vi "SRRead.vi"(8 "error in (no error)":errorcluster, 11 "Data In":T1) -> (0 "error out":errorcluster, 1 "BarCodeRead":string="TH-55ES630W,%71234567,4717523005417\r", 3 "Data Out":T1)   [LabVIEW 2014]
uses:
  controls/Data.ctl
panel:
  out "Boolean":bool
  # "日期"
  # "機種名稱"
  # "機種代號"
  # "商品條碼"
  # "台"
  # "OK"
  # "NG"
  # "台"
  # "總計"
  # "台"
  # "日期"
  # "機種名稱"
  # "機種代號"
  # "商品條碼"
  # "台"
  # "OK"
  # "NG"
  # "台"
  # "總計"
  # "台"
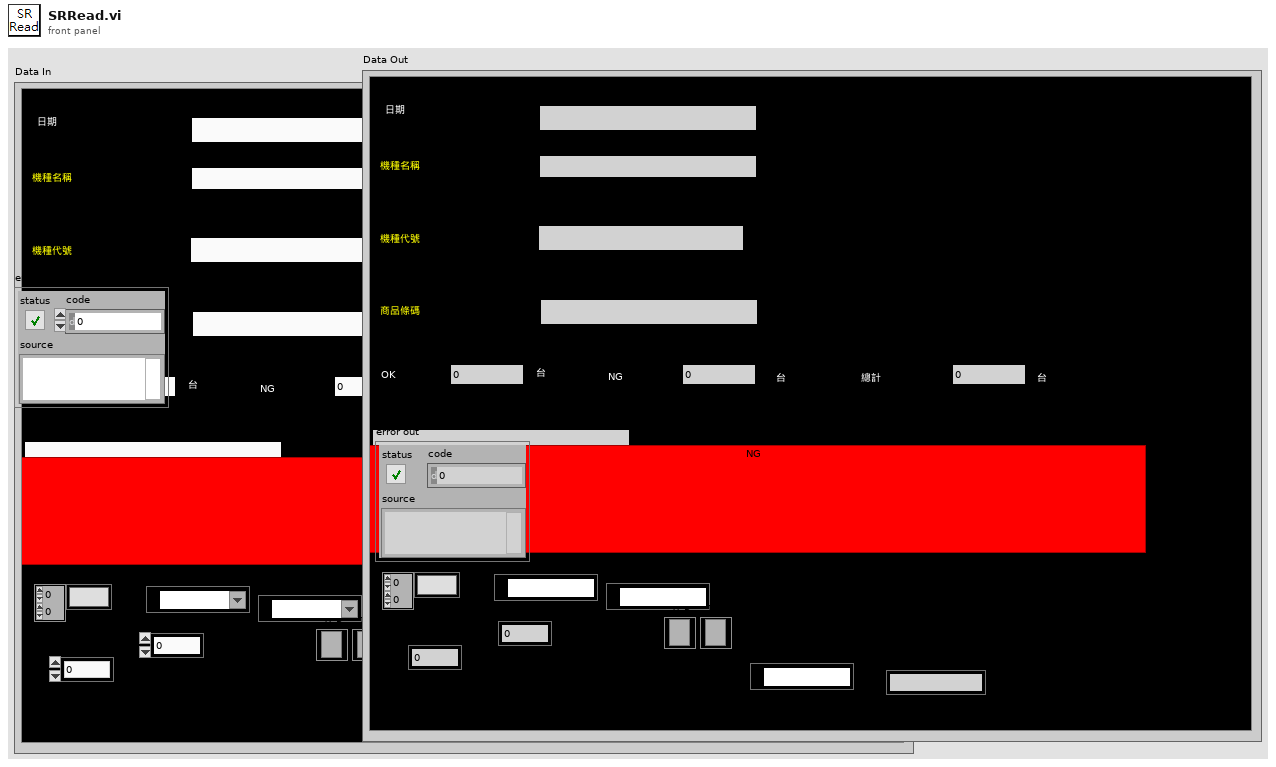
[diagram p1: front panel]
types:
  T1 = typedef "Data.ctl" = cluster{"Date":string, "BarCode1":string, "BarCode2":string, "BarCode3":string, "Message":string, "OK Count":u16, "NG Count":u16, "Total Count":u16, "ModelData":string[][], "OK&NG":bool, "COM1":refnum<visa-resource-name>, "COM2":refnum<visa-resource-name>, "IO":i32, "Time":u32, "TCP":refnum<k5>, "TCP 2":refnum<k5>, "COM3":refnum<visa-resource-name>, "CheckPars":string}
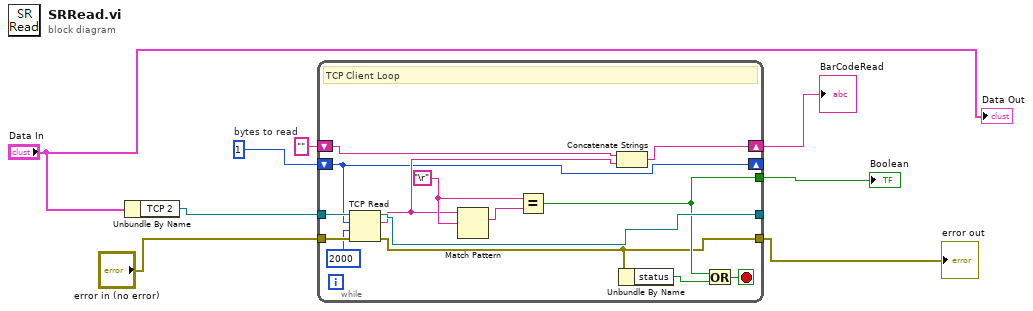
[diagram p0: block diagram]
diagram:
  w8 = 1  # bytes to read
  n1 = Unbundle By Name("Data In") -> ("TCP 2"=w4:refnum<k5>)
  n2 = while {
    tunnel: "error in (no error)" -> [w21]
    tunnel: w4 -> [w22]
    tunnel: [w16] -> _
    tunnel: [w10] -> w2
    shift-right: [w11] -> _
    shift-left: w8 -> [w11]
    tunnel: [w15] -> w7
    shift-right: [w13] -> w5
    shift-left: "" -> [w12]
    stop <- w20 stop-if-true
    w17 = "\r"
    # "TCP Client Loop"
    n3 = TCP Read(connection ID=w22, bytes to read=w11, error in (no error)=w21, 9:2000 ("timeout ms (25000)")) -> (connection ID out=w16:refnum<k5>, data out=w14:string, error out=w10:errorcluster)  [unwired: 1 in]
    n4 = Match Pattern(string=w14, regular expression=w17) -> (match substring=w18:string)  [unwired: 1 in, 3 out]
    n5 = Equal?(x=w17, y=w18) -> (x = y?=w15:bool)
    n6 = Concatenate Strings(w12, w14) -> (w13:string)
    n7 = Unbundle By Name(w10) -> ("status"=w9:bool)
    n8 = Or(x=w15, y=w9) -> (x .or. y?=w20:bool)
  }
  "Boolean" <- w7
  "BarCodeRead" <- w5
  "error out" <- w2
  "Data Out" <- "Data In"
